vi "Disconnect All.vi"(8 "error in (no error)":errorcluster, 11 "PIPXI40 Matrix in":refnum<class "PIPXI40 Matrix.lvclass">) -> (0 "error out":errorcluster, 3 "PIPXI40 Matrix out":refnum<class "PIPXI40 Matrix.lvclass">)   [LabVIEW 2020, in "PIPXI40.lvlib" / "PIPXI40 Matrix.lvclass"]
uses:
  PIPXI40 Matrix.lvclass
  D:/WSGitHub/RTFWK/Realization/PIPXI40 Base/PIPXI40 Base.lvclass
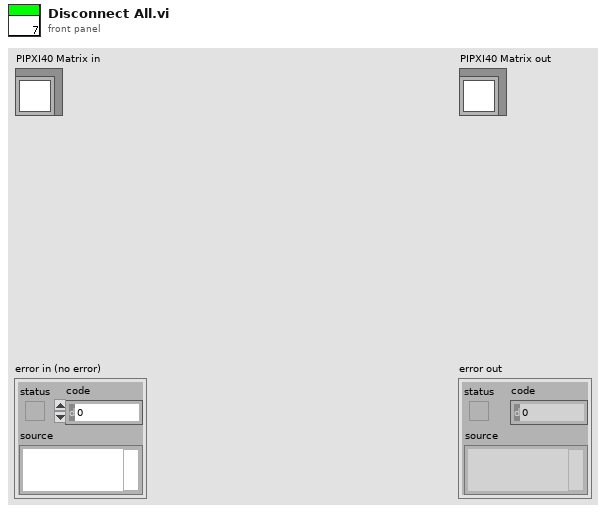
[diagram p1: front panel]
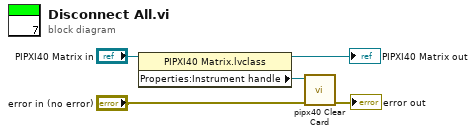
[diagram p0: block diagram]
diagram:
  n1 = property class="PIPXI40 Matrix.lvclass"(reference="PIPXI40 Matrix in") -> (reference out=→"PIPXI40 Matrix out":refnum<class "PIPXI40 Matrix.lvclass">, "Properties:Instrument handle"=w5:refnum<visa-resource-name>)  [unwired: 1 in, 1 out]
  n2 = call <instrlib>:"pipx40 Clear Card.vi"("error in (no error)"="error in (no error)", "instrument handle"=w5) -> ("error out"=→"error out":errorcluster)  [unwired: 8 in, 1 out]
